vi "Format.vi"(7 "Max Errors":bool, 10 "MultiErrors":T1[](array[typedef]), 11 "MultiError Formatter in":refnum<class "MultiError Formatter.lvclass">) -> (0 "error out":errorcluster)   [LabVIEW 2020, in "VolatusErrorUtilities.lvlib" / "MultiError Formatter.lvclass"]
uses:
  MultiError Formatter.lvclass
  MultiError.ctl
  VolatusErrorUtilities.lvlib
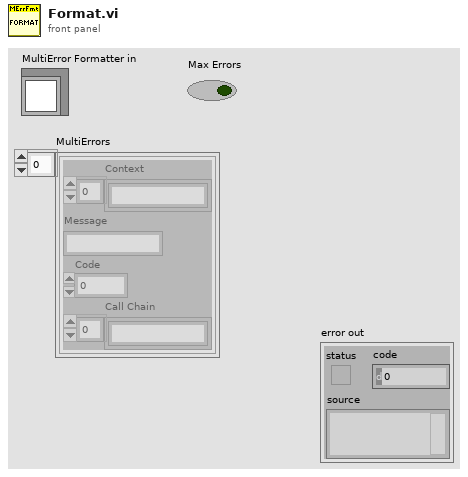
[diagram p1: front panel]
types:
  T1 = typedef "VolatusErrorUtilities.lvlib/MultiError.ctl" = cluster{"Context":string[], "Message":string, "Code":i32, "Call Chain":string[]}
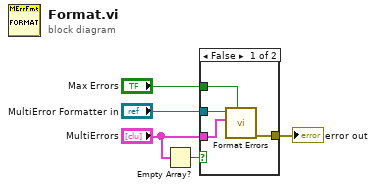
[diagram p0: block diagram]
diagram:
  n1 = Empty Array?(array="MultiErrors") -> (empty?=w5:bool)
  n2 = case shown="False" w5 {
    tunnel: "MultiErrors" -> [w7 _]
    tunnel: "MultiError Formatter in" -> [w9 _]
    tunnel: "Max Errors" -> [w8 _]
    tunnel: [w6 _] -> w1
    frame False {
      n3 = call-dynamic "Format Errors.vi"("Max Errors"=w8, "MultiErrors"=w7, "MultiError Formatter in"=w9) -> ("error out"=w6:errorcluster)  [unwired: 8 in]
    }
    frame True {
    }
  }
  "error out" <- w1
